vi "Map Tags to Channels.vi"(7 "instance id":string, 8 "error in (no error)":errorcluster, 9 "String Array":string[][](array[string]), 10 "Lines":T1[](array[typedef]), 11 "engine configuration in":refnum<class "engine configuration.lvclass">) -> (0 "error out":errorcluster, 3 "engine configuration out":refnum<class "engine configuration.lvclass">)   [LabVIEW 2014, in "UI Reference editor node.lvclass"]
uses:
  UI Reference editor node.lvclass
  module/configuration/Line.ctl
  <vilib>/NI/Tag Bus Module Framework/channel/TBM channel.lvclass
  <vilib>/NI/Module Execution Interface/Engine Configuration/engine configuration.lvclass
  <vilib>/NI/Tag Bus/tag/tag descriptor.lvclass/tag descriptor.ctl
  <vilib>/NI/Tag Bus/tag/tag descriptor.lvclass
  module/configuration/UI Reference configuration.lvclass
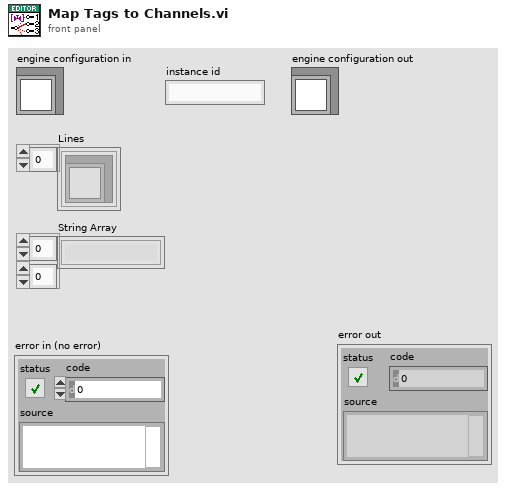
[diagram p1: front panel]
types:
  T1 = typedef "UI Reference configuration.lvclass/Line.ctl" = cluster{"channel":refnum<class "TBM channel.lvclass">}
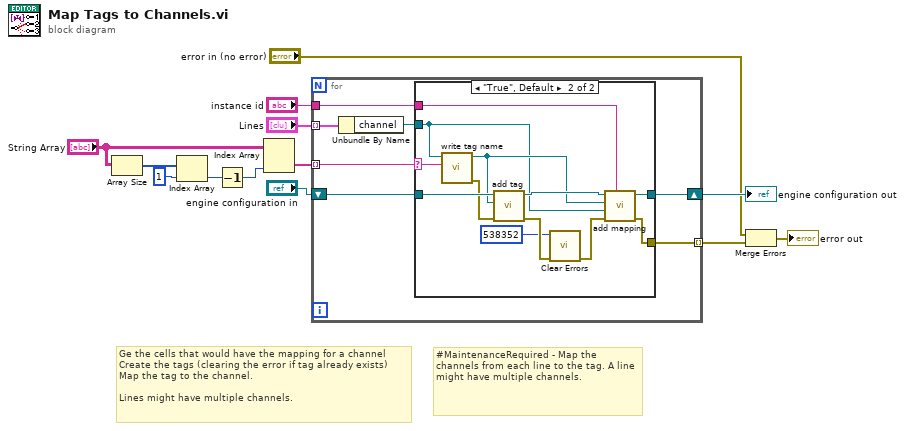
[diagram p0: block diagram]
diagram:
  # "#MaintenanceRequired - Map the channels from each line to the tag. A line might have multiple channels."
  # "Ge the cells that would have the mapping for a channel\nCreate the tags (clearing the error if tag already exists) \nMap the tag to the channel.\n\nLines might have multiple channels."
  n1 = Array Size(array="String Array") -> (size(s)=w8:i32[])
  n2 = Index Array(array=w8, index=1) -> (element=w6:i32)
  n3 = Decrement(x=w6) -> (x-1=w5:i32)
  n4 = Index Array(array="String Array", index (col)=w5) -> (element=w3:string[])  [unwired: 1 in]
  n5 = for {
    tunnel: "Lines" -> [w20] mode=indexing
    tunnel: w3 -> [w14] mode=indexing
    shift-right: [w19] -> w10
    shift-left: "engine configuration in" -> [w16]
    tunnel: "instance id" -> [w18]
    tunnel: [w17] -> w12 mode=indexing
    n6 = Unbundle By Name(w20) -> ("channel"=w15:refnum<class "TBM channel.lvclass">)
    n7 = case shown="\"True\", Default" w14 {
      selector: w14 -> [_ w22]
      tunnel: [w21 w33] -> w19
      tunnel: w18 -> [_ w32]
      tunnel: [_ w31] -> w17
      tunnel: w16 -> [w21 w30]
      tunnel: w15 -> [_ w27]
      frame "" {
      }
      frame "True", Default {
        n8 = call <vilib>:"write tag name.vi"("name"=w22, "system tag in"=w27) -> ("error out"=w26:errorcluster, "system tag out"=w28:refnum<class "TBM channel.lvclass">)  [unwired: 8 in]
        n9 = call-dynamic "add tag.vi"("error in"=w26, "tag descriptor"=w28, "engine configuration in"=w30) -> ("error out"=w25:errorcluster, "engine configuration out"=w29:refnum<class "engine configuration.lvclass">)  [unwired: 7 in]
        n10 = call <vilib>:"Clear Errors.vi"("error in (no error)"=w25, "specific error code to clear (0: all)"=538352) -> ("error out"=w24:errorcluster)  [unwired: 4 in, 1 out]
        n11 = call-dynamic "add mapping.vi"("owner ID"=w32, "error in"=w24, "channel"=w27, "tag descriptor"=w28, "engine configuration"=w29) -> ("error out"=w31:errorcluster, "engine configuration out"=w33:refnum<class "engine configuration.lvclass">)  [unwired: 5 in]
      }
    }
  }
  "engine configuration out" <- w10
  n12 = Merge Errors("error in (no error)", w12) -> (→"error out":errorcluster)
